vi "Get Step Config.vi"(0 "VI In":refnum<vi>, 11 "error in":errorcluster) -> (4 "VI out":refnum<vi>, 6 "Wash Array":T1[](array[typedef]), 15 "error out":errorcluster)   [LabVIEW 2016]
uses:
  Controls/Wash Step Config.ctl
  <vilib>/Utility/config.llb/NI_LVConfig.lvlib
  <vilib>/Utility/config.llb/Read Key (Double).vi
  <vilib>/Utility/config.llb/Read Key (U32).vi
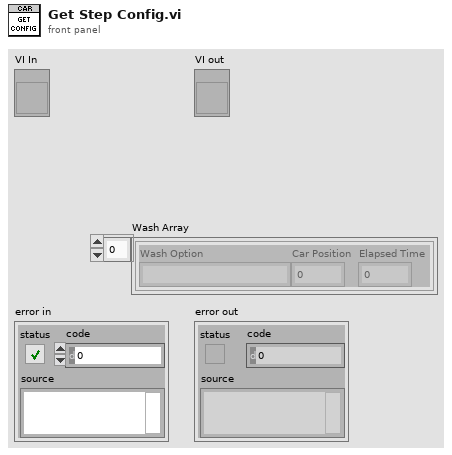
[diagram p1: front panel]
types:
  T1 = typedef "Wash Step Config.ctl" = cluster{"Wash Option":string, "Car Position":i32, "Elapsed Time":dbl}
  T2 = typedef "NI_LVConfig.lvlib/Config Data RefNum.ctl" = refnum<k1>
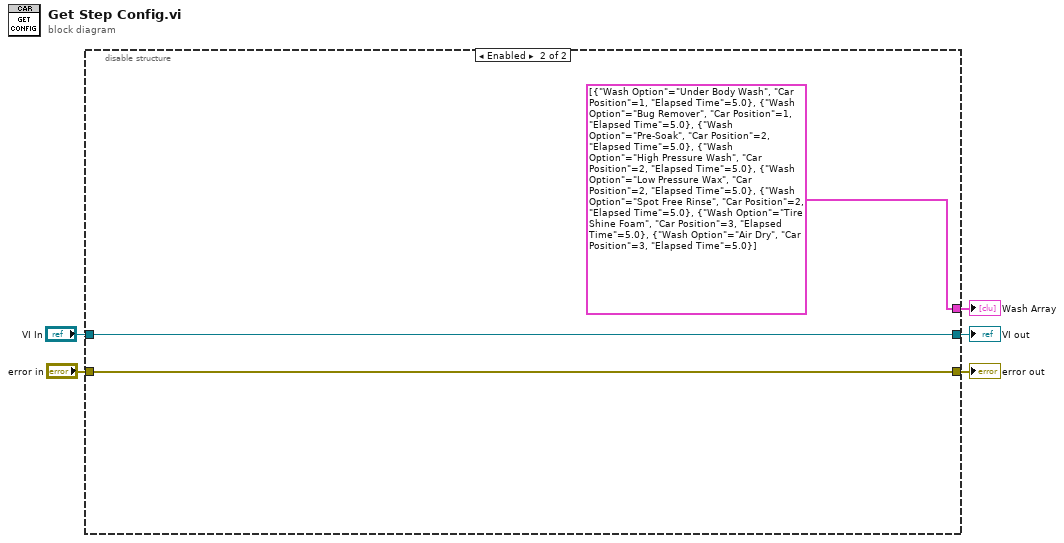
[diagram p0: block diagram]
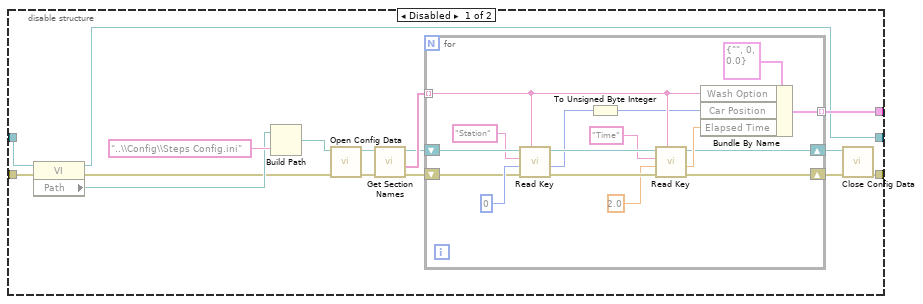
[diagram p2: hidden frame]
diagram:
  n1 = disable-structure shown="Enabled" {
    disable-tunnel: [w21 T1[] [{"Wash Option"="Under Body Wash", "Car Position"=1, "Elapsed Time"=5.0}, {"Wash Option"="Bug Remover", "Car Position"=1, "Elapsed Time"=5.0}, {"Wash Option"="Pre-Soak", "Car Position"=2, "Elapsed Time"=5.0}, {"Wash Option"="High Pressure Wash", "Car Position"=2, "Elapsed Time"=5.0}, {"Wash Option"="Low Pressure Wax", "Car Position"=2, "Elapsed Time"=5.0}, {"Wash Option"="Spot Free Rinse", "Car Position"=2, "Elapsed Time"=5.0}, {"Wash Option"="Tire Shine Foam", "Car Position"=3, "Elapsed Time"=5.0}, {"Wash Option"="Air Dry", "Car Position"=3, "Elapsed Time"=5.0}] ("Wash Array")] -> w5
    disable-tunnel: [w20 w39] -> w4
    disable-tunnel: "VI In" -> [w19 w40]
    disable-tunnel: "error in" -> [w18 w39]
    disable-tunnel: [w17 w40] -> w1
    frame Disabled {
      n2 = property class="VI"(reference=w19, error in=w18) -> (reference out=w17:refnum<vi>, error out=w6:errorcluster, "Path"=w7:path)
      n3 = Build Path(base path=w7, name or relative path="..\\Config\\Steps Config.ini") -> (appended path=w9:path)
      n4 = call <vilib>:"Open Config Data.vi"("error in (no error)"=w6, "configuration file path"=w9) -> ("error out"=w11:errorcluster, "refnum"=w10:T2)  [unwired: 7 in, 1 out]
      n5 = call <vilib>:"Get Section Names.vi"("error in (no error)"=w11, "refnum"=w10) -> ("error out"=w14:errorcluster, "section names"=w13:string[], "refnum out"=w12:T2)  [unwired: 7 in]
      n6 = for {
        tunnel: w13 -> [w30] mode=indexing
        tunnel: [w26] -> w21 mode=indexing
        shift-right: [w25] -> w15
        shift-left: w14 -> [w34]
        shift-right: [w24] -> w16
        shift-left: w12 -> [w36]
        n7 = call-poly <vilib>:"Read Key.vi"("section"=w30, "error in (no error)"=w34, "default value"=u32 0, "key"="Station", "refnum"=w36) -> ("error out"=w32:errorcluster, "value"=w29:u32, "refnum out"=w33:T2)  [unwired: 3 in, 1 out]
        n8 = To Unsigned Byte Integer(number=w29) -> (unsigned 8bit integer=w27:u8)
        n9 = call-poly <vilib>:"Read Key.vi"("section"=w30, "error in (no error)"=w32, "default value"=2.0, "key"="Time", "refnum"=w33) -> ("error out"=w25:errorcluster, "value"=w28:dbl, "refnum out"=w24:T2)  [unwired: 3 in, 1 out]
        n10 = Bundle By Name(cluster=T1 {"Wash Option"="", "Car Position"=0, "Elapsed Time"=0.0}, "Wash Option"=w30, "Car Position"=w27, "Elapsed Time"=w28) -> (w26:T1)
      }
      n11 = call <vilib>:"Close Config Data.vi"("error in (no error)"=w15, "refnum"=w16) -> ("error out"=w20:errorcluster)  [unwired: 8 in, 1 out]
    }
    frame Enabled {
    }
  }
  "Wash Array" <- w5
  "error out" <- w4
  "VI out" <- w1
